vi "Maxi Gauge-RW Sensor On-Off.vi"(0 "VISA-Ressource in":refnum<visa-resource-name>, 1 "Sensor 1 Set":i8(ring) items=["no change", "off", "on"], 2 "Sensor 2 Set":i8(ring) items=["no change", "off", "on"], 3 "Sensor 3 Set":i8(ring) items=["no change", "off", "on"], 4 "Sensor 4 Set":i8(ring) items=["no change", "off", "on"], 5 "Fehler (Eingang)":errorcluster, 6 "Node address":i8=-1 min=-1 max=31 step=1, 7 "Sensor 5 Set":i8(ring) items=["no change", "off", "on"], 8 "W/R":bool, 9 "Sensor 6 Set":i8(ring) items=["no change", "off", "on"], 10 "No ON/OFF ID´s":string[](array[string])=["no Sensor", "APR/ACR", "TPR"]) -> (11 "Sensor 6 Get":i8(ring)=1 items=["no change", "off", "on"], 13 "Sensor 5 Get":i8(ring)=1 items=["no change", "off", "on"], 14 "VISA-Ressource out":refnum<visa-resource-name>, 15 "Sensor 1 Get":i8(ring)=1 items=["no change", "off", "on"], 16 "Sensor 2 Get":i8(ring)=1 items=["no change", "off", "on"], 17 "Sensor 3 Get":i8(ring)=1 items=["no change", "off", "on"], 18 "Sensor 4 Get":i8(ring)=1 items=["no change", "off", "on"], 19 "Fehler (Ausgang)":errorcluster)   [LabVIEW 2013, in "Maxi Gauge.lvlib"]
uses:
  <instrlib>/Maxi Gauge/Maxi Gauge.lvlib
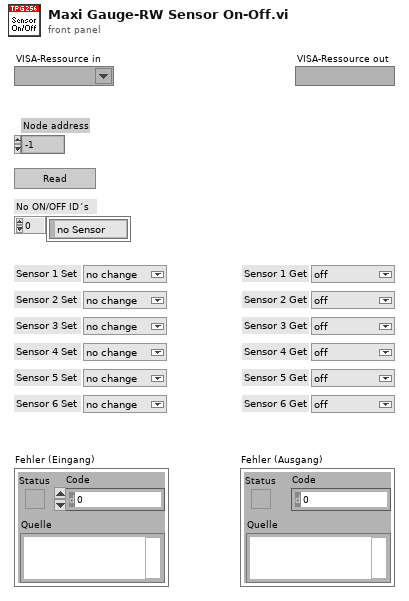
[diagram p1: front panel]
types:
  T1 = cluster{"Sensor 1":string, "Sensor 2":string, "Sensor 3":string, "Sensor 4":string, "Sensor 5":string, "Sensor 6":string}
  T2 = cluster{"[0]":i16, "[1]":i16, "[2]":i16, "[3]":i16, "[4]":i16, "[5]":i16}
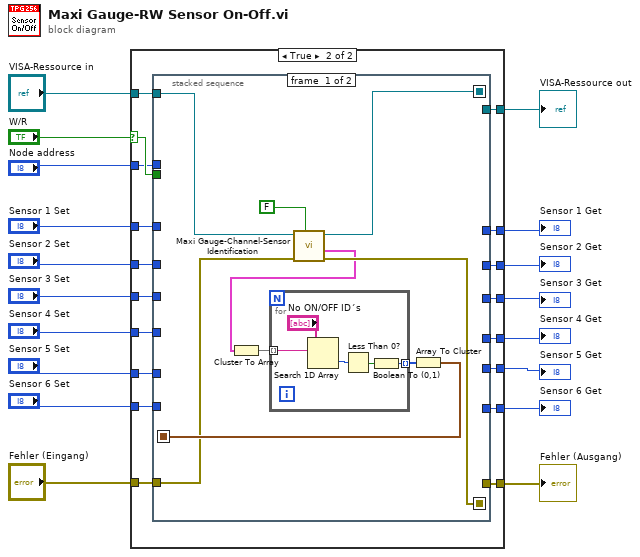
[diagram p0: block diagram]
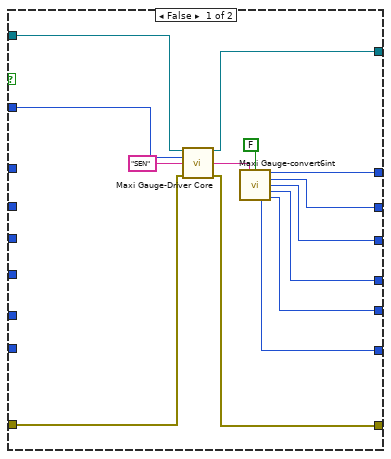
[diagram p2: hidden frame]
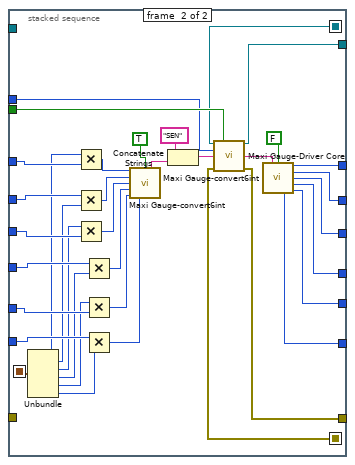
[diagram p3: hidden frame]
diagram:
  n1 = case shown="True" "W/R" {
    selector: "W/R" -> [_ w50]
    tunnel: [w32 w43] -> w5
    tunnel: [w31 w44] -> w6
    tunnel: [w30 w45] -> w7
    tunnel: [w29 w46] -> w8
    tunnel: [w28 w47] -> w9
    tunnel: [w27 w48] -> w10
    tunnel: "Sensor 6 Set" -> [_ w37]
    tunnel: "Sensor 5 Set" -> [_ w38]
    tunnel: "Sensor 4 Set" -> [_ w39]
    tunnel: "Sensor 3 Set" -> [_ w40]
    tunnel: "Sensor 2 Set" -> [_ w41]
    tunnel: "Sensor 1 Set" -> [_ w42]
    tunnel: "Node address" -> [w24 w49]
    tunnel: "VISA-Ressource in" -> [w22 w36]
    tunnel: [w21 w35] -> w3
    tunnel: "Fehler (Eingang)" -> [w20 w34]
    tunnel: [w19 w33] -> w1
    frame False {
      n2 = call <instrlib>:"Maxi Gauge-Driver Core.vi"("VISA-Ressource in"=w22, "Node address"=w24, "Command"="SEN", "Fehler (Eingang)"=w20) -> ("VISA-Ressource out"=w21:refnum<visa-resource-name>, "String Out"=w26:string, "Fehler (Ausgang)"=w19:errorcluster)  [unwired: 9 in]
      n3 = call <instrlib>:"Maxi Gauge-convert6int.vi"("String in"=w26, "W/R [W: Int in; Str out ]"=FALSE) -> ("Integer1 out"=w27:u8, "Integer2 out"=w28:u8, "Integer3 out"=w29:u8, "Integer4 out"=w30:u8, "Integer6 out"=w32:u8, "Integer5 out"=w31:u8)  [unwired: 7 in, 1 out]
    }
    frame True {
      n4 = stacked-sequence {
        seq-local: [w56 _] -> [_ w76]
        seq-local: [w54 _] -> [_ w68]
        seq-local: [w52 _] -> [_ w66]
        tunnel: w50 -> [_ w99]
        tunnel: w49 -> [_ w98]
        tunnel: [_ w97] -> w48
        tunnel: [_ w96] -> w47
        tunnel: [_ w95] -> w46
        tunnel: [_ w94] -> w45
        tunnel: [_ w93] -> w44
        tunnel: [_ w92] -> w43
        tunnel: w42 -> [_ w90]
        tunnel: w41 -> [_ w89]
        tunnel: w40 -> [_ w88]
        tunnel: w39 -> [_ w87]
        tunnel: w38 -> [_ w86]
        tunnel: w37 -> [_ w85]
        tunnel: w36 -> [w55 _]
        tunnel: [_ w67] -> w35
        tunnel: w34 -> [w53 _]
        tunnel: [_ w65] -> w33
        frame #0 {
          n5 = call <instrlib>:"Maxi Gauge-Channel-Sensor Identification.vi"("W/R"=FALSE, "Fehler (Eingang, kein Fehler)"=w53, "VISA-Ressource in"=w55) -> ("Fehler (Ausgang)"=w52:errorcluster, "Get Sensor Identification"=w51:T1, "VISA-Ressource out"=w54:refnum<visa-resource-name>)  [unwired: 5 in, 1 out]
          n6 = Cluster To Array(cluster=w51) -> (array=w59:string[])
          n7 = for {
            tunnel: w59 -> [w60] mode=indexing
            tunnel: [w62] -> w57 mode=indexing
            n8 = Search 1D Array(1D array="No ON/OFF ID´s", element=w60) -> (index of element=w64:i32)  [unwired: 1 in]
            n9 = Less Than 0?(x=w64) -> (x < 0?=w63:bool)
            n10 = Boolean To (0,1)(Boolean=w63) -> (0, 1=w62:i16)
          }
          n11 = Array To Cluster(array=w57) -> (cluster=w56:T2)
        }
        frame #1 {
          n12 = Unbundle(w76) -> ("[0]"=w75:i16, "[1]"=w74:i16, "[2]"=w73:i16, "[3]"=w72:i16, "[4]"=w71:i16, "[5]"=w70:i16)
          n13 = Multiply(x=w75, y=w90) -> (x*y=w82:i16)
          n14 = Multiply(x=w89, y=w74) -> (x*y=w81:i16)
          n15 = Multiply(x=w73, y=w88) -> (x*y=w80:i16)
          n16 = Multiply(x=w87, y=w72) -> (x*y=w79:i16)
          n17 = Multiply(x=w71, y=w86) -> (x*y=w78:i16)
          n18 = Multiply(x=w85, y=w70) -> (x*y=w77:i16)
          n19 = call <instrlib>:"Maxi Gauge-convert6int.vi"("Integer1 in"=w82, "W/R [W: Int in; Str out ]"=TRUE, "Integer2 in"=w81, "Integer3 in"=w80, "Integer4 in"=w79, "Integer5 in"=w78, "Integer6 in"=w77) -> ("String out"=w83:string)  [unwired: 2 in, 6 out]
          n20 = Concatenate Strings("SEN", w83) -> (w69:string)
          n21 = call <instrlib>:"Maxi Gauge-Driver Core.vi"("VISA-Ressource in"=w68, "Write/Read"=w99, "Node address"=w98, "Command"=w69, "Fehler (Eingang)"=w66) -> ("VISA-Ressource out"=w67:refnum<visa-resource-name>, "String Out"=w101:string, "Fehler (Ausgang)"=w65:errorcluster)  [unwired: 8 in]
          n22 = call <instrlib>:"Maxi Gauge-convert6int.vi"("String in"=w101, "W/R [W: Int in; Str out ]"=FALSE) -> ("Integer1 out"=w97:u8, "Integer2 out"=w96:u8, "Integer3 out"=w95:u8, "Integer4 out"=w94:u8, "Integer6 out"=w92:u8, "Integer5 out"=w93:u8)  [unwired: 7 in, 1 out]
        }
      }
    }
  }
  "Sensor 1 Get" <- w10
  "Sensor 2 Get" <- w9
  "Sensor 3 Get" <- w8
  "Sensor 4 Get" <- w7
  "Sensor 5 Get" <- w6
  "Sensor 6 Get" <- w5
  "VISA-Ressource out" <- w3
  "Fehler (Ausgang)" <- w1
